vi "From LabVIEW.vi"(4 "BB Players Map in":refnum<class "BB Players Map.lvclass">, 8 "error in (no error)":errorcluster, 10 "Value":refnum<class>) -> (0 "error out":errorcluster, 2 "DbRow":variant)   [LabVIEW 2020, in "ORM_Examples.lvlib" / "BB Players Map.lvclass"]
doc: "This converts the private data of the bbPlayers class to a \"DbRow\" structure. This is a \"dictionary\" in LabVIEW implemented as variant attribute name:value pairs."
uses:
  BB Players Map.lvclass
  C:/Program Files/National Instruments/LabVIEW 2020/vi.lib/Viviota/shared/ORM.lvlibp/ORM/TypeMap/TypeMap.lvclass
  BB Players/bbPlayers.lvclass
  <vilib>/Viviota/shared/ORM.lvlibp/ORM/TypeMap/Read Autokey.vi
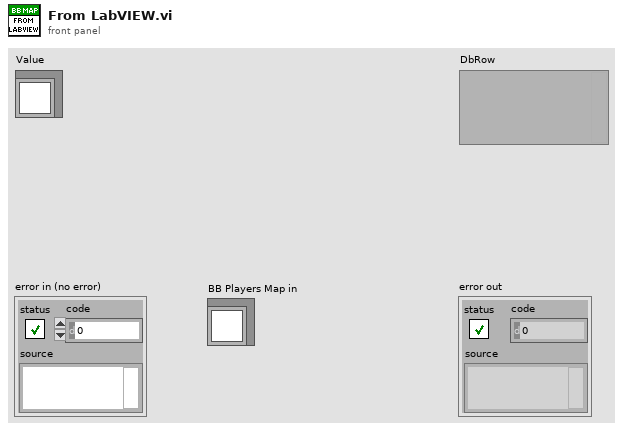
[diagram p1: front panel]
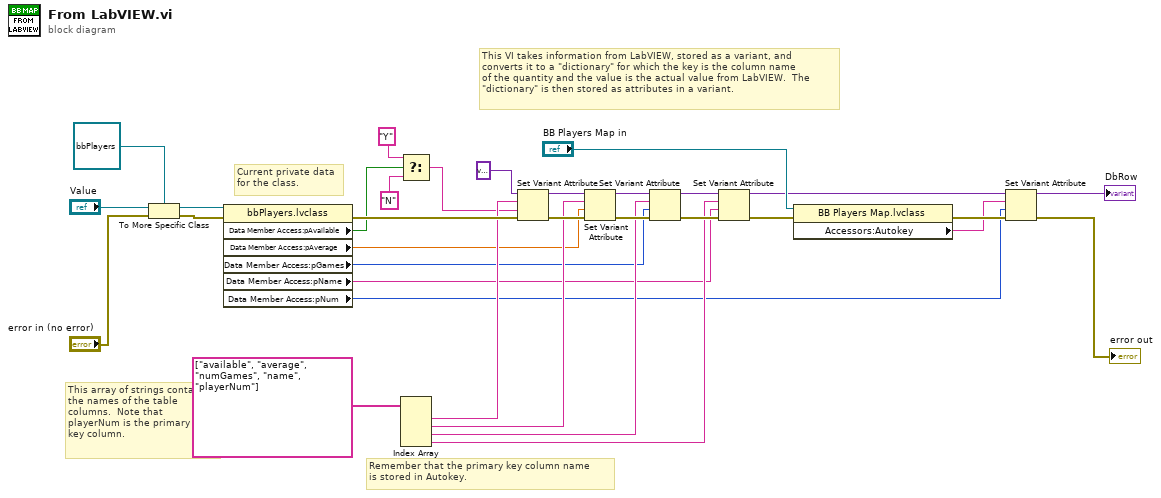
[diagram p0: block diagram]
diagram:
  # "Remember that the primary key column name\nis stored in Autokey."
  # "Current private data\nfor the class."
  # "This array of strings contains\nthe names of the table\ncolumns.  Note that \nplayerNum is the primary\nkey column."
  # "This VI takes information from LabVIEW, stored as a variant, and\nconverts it to a \"dictionary\" for which the key is the column name\nof the quantity and the value is the actual value from LabVIEW.  The\n\"dictionary\" is then stored as attributes in a variant."
  n1 = To More Specific Class(target class=refnum<class "bbPlayers.lvclass"> refnum ("bbPlayers.lvclass"), reference="Value", error in="error in (no error)") -> (specific class reference=w30:refnum<class "bbPlayers.lvclass">, error out=w29:errorcluster)
  n2 = property class="bbPlayers.lvclass"(reference=w30, error in=w29) -> (error out=w27:errorcluster, "Data Member Access:pAvailable"=w13:bool, "Data Member Access:pAverage"=w7:dbl, "Data Member Access:pGames"=w5:i32, "Data Member Access:pName"=w3:string, "Data Member Access:pNum"=w1:i32)  [unwired: 1 out]
  n3 = Select(t="Y", s=w13, f="N") -> (s? t:f=w9:string)
  n4 = Index Array(array=string[] ["available", "average", "numGames", "name", "playerNum"]) -> (element #1=w10:string, element #2=w8:string, element #3=w6:string, element #4=w4:string)  [unwired: 4 in]
  n5 = Set Variant Attribute(Variant=variant ("Value"), name=w10, value=w9, error in=w27) -> (Variant out=w22:variant, error out=w26:errorcluster)  [unwired: 1 out]
  n6 = Set Variant Attribute(Variant=w22, name=w8, value=w7, error in=w26) -> (Variant out=w21:variant, error out=w25:errorcluster)  [unwired: 1 out]
  n7 = Set Variant Attribute(Variant=w21, name=w6, value=w5, error in=w25) -> (Variant out=w20:variant, error out=w24:errorcluster)  [unwired: 1 out]
  n8 = Set Variant Attribute(Variant=w20, name=w4, value=w3, error in=w24) -> (Variant out=w16:variant, error out=w19:errorcluster)  [unwired: 1 out]
  n9 = property class="BB Players Map.lvclass"(reference="BB Players Map in", error in=w19) -> (error out=w17:errorcluster, "Accessors:Autokey"=w2:string)  [unwired: 1 out]
  n10 = Set Variant Attribute(Variant=w16, name=w2, value=w1, error in=w17) -> (Variant out=→"DbRow":variant, error out=→"error out":errorcluster)  [unwired: 1 out]
